vi "Show Tables.vi"(8 "error in (no error)":errorcluster, 10 "Report Data.Schema":string, 11 "Import Export in":refnum<class "Export.lvclass">) -> (0 "error out":errorcluster, 3 "Import Export out":refnum<class "Export.lvclass">)   [LabVIEW 2023, in "Data Analysis.lvlib" / "Export.lvlib" / "Export.lvclass"]
uses:
  Export.lvclass
  Export.lvclass/Export.ctl
  HardwareAbstractionLayer_LVOOP/Database/Database.lvclass
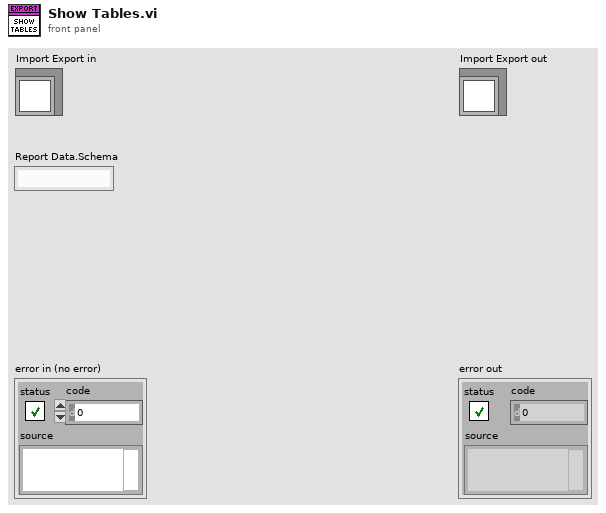
[diagram p1: front panel]
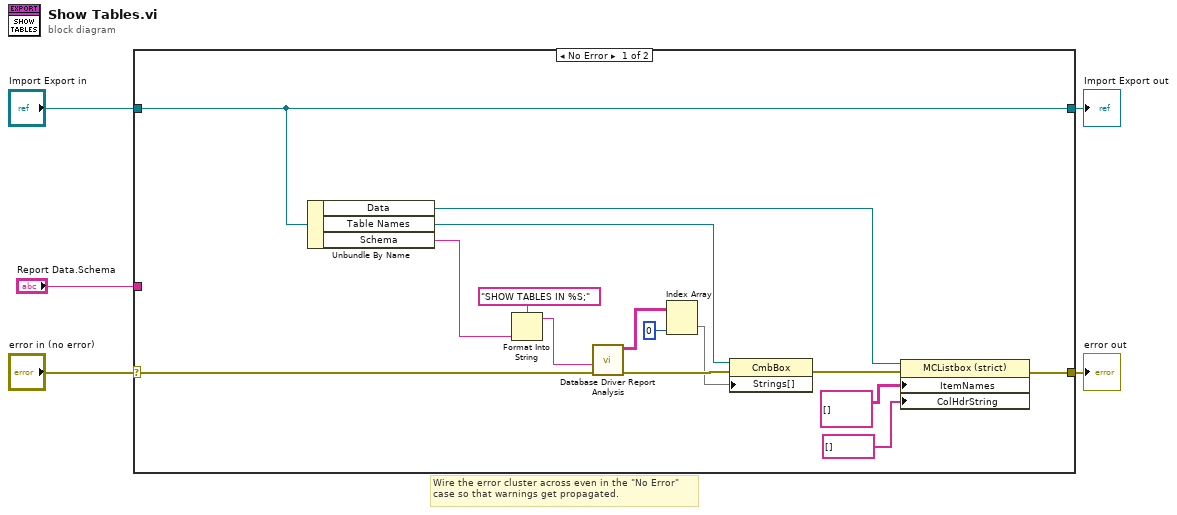
[diagram p0: block diagram]
diagram:
  # "Wire the error cluster across even in the \"No Error\"\ncase so that warnings get propagated."
  n1 = case shown="No Error" "error in (no error)" {
    selector: "error in (no error)" -> [w16 w22]
    tunnel: [w17 w22] -> w4
    tunnel: [w6 w21] -> w2
    tunnel: "Import Export in" -> [w6 w21]
    tunnel: "Report Data.Schema" -> [_ _]
    frame No Error {
      n2 = Unbundle By Name(w6) -> ("Data"=w20:refnum<vi>, "Table Names"=w10:refnum<vi>, "Schema"=w14:string)
      n3 = Format Into String(format string="SHOW TABLES IN %S;", w14) -> (resulting string=w13:string)  [unwired: 2 in, 1 out]
      n4 = call "Database Driver Report Analysis.vi"("error in"=w16, "SQL query"=w13) -> ("error out"=w9:errorcluster, "data"=w12:string[][])  [unwired: 6 in, 2 out]
      n5 = Index Array(array=w12, index (col)=0 ("disabled index (col)")) -> (element=w7:string[])  [unwired: 1 in]
      n6 = property class="CmbBox"(reference=w10, error in=w9, "Strings[]"=w7) -> (error out=w8:errorcluster)  [unwired: 1 out]
      n7 = property class="MCListbox (strict)"(reference=w20, error in=w8, "ItemNames"=string[][] [] ("Item Names"), "ColHdrString"=string[] [] ("Column Header Strings[]")) -> (error out=w17:errorcluster)  [unwired: 1 out]
    }
    frame Error {
    }
  }
  "error out" <- w4
  "Import Export out" <- w2
